vi "Convert From Base64.vi"(8 "error in (no error)":errorcluster, 11 "Base64 String":string) -> (0 "error out":errorcluster, 3 "String":string)   [LabVIEW 2015, in "Front Panel Publisher.lvlib"]
doc: "This VI converts a Base 64 string to its string equivalent. Base64 strings are commonly used in Internet protocols such as HTTP, SMTP, etc."
uses:
  Front Panel Publisher.lvlib
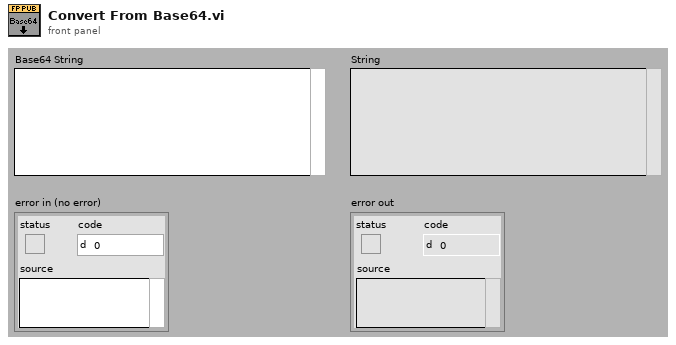
[diagram p1: front panel]
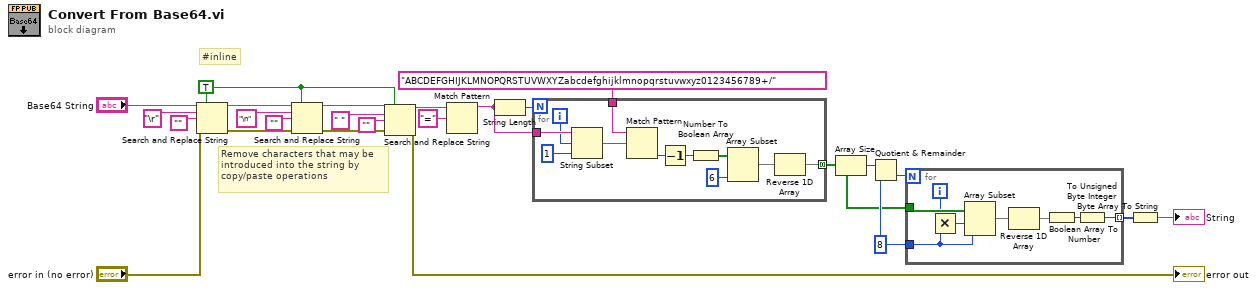
[diagram p0: block diagram]
diagram:
  w25 = TRUE ("replace all? (F)")
  w14 = 8 ("y")
  # "#inline"
  # "Remove characters that may be\nintroduced into the string by\ncopy/paste operations"
  n1 = Search and Replace String(replace all?=w25, input string="Base64 String", search string="\r" ("replace string (\"\")"), replace string="", error in="error in (no error)") -> (result string=w19:string, error out=w6:errorcluster)  [unwired: 5 out]
  n2 = Search and Replace String(replace all?=w25, input string=w19, search string="\n" ("replace string (\"\")"), replace string="", error in=w6) -> (result string=w23:string, error out=w5:errorcluster)  [unwired: 5 out]
  n3 = Search and Replace String(replace all?=w25, input string=w23, search string=" " ("replace string (\"\")"), replace string="", error in=w5) -> (result string=w24:string, error out=→"error out":errorcluster)  [unwired: 5 out]
  n4 = Match Pattern(string=w24, regular expression="=") -> (before substring=w9:string)  [unwired: 4 out]
  n5 = String Length(string=w9) -> (length=w7:i32)
  n6 = for {
    N: w7 -> [_]
    tunnel: w9 -> [w36]
    tunnel: "ABCDEFGHIJKLMNOPQRSTUVWXYZabcdefghijklmnopqrstuvwxyz0123456789+/" -> [w33]
    tunnel: [w26] -> w13 mode=concatenating
    i -> [w34]
    n7 = String Subset(string=w36, offset (0)=w34, length (rest)=1 ("length (rest)")) -> (substring=w32:string)
    n8 = Match Pattern(string=w33, regular expression=w32) -> (offset past match=w31:i32)  [unwired: 4 out]
    n9 = Decrement(x=w31) -> (x-1=w30:i32)
    n10 = Number To Boolean Array(number=w30) -> (Boolean array=w29:bool[])
    n11 = Array Subset(array=w29, length=6) -> (w27:bool[])  [unwired: 1 in]
    n12 = Reverse 1D Array(array=w27) -> (reversed array=w26:bool[])
  }
  n13 = Array Size(array=w13) -> (size(s)=w11:i32)
  n14 = Quotient & Remainder(x=w11, y=w14) -> (floor(x/y)=w12:i32)  [unwired: 1 out]
  n15 = for {
    N: w12 -> [_]
    tunnel: w13 -> [w44]
    tunnel: w14 -> [w43]
    tunnel: [w39] -> w15 mode=indexing
    i -> [w42]
    n16 = Multiply(x=w42, y=w43) -> (x*y=w37:i32)
    n17 = Array Subset(array=w44, index=w37, length=w43) -> (w41:bool[])
    n18 = Reverse 1D Array(array=w41) -> (reversed array=w38:bool[])
    n19 = Boolean Array To Number(Boolean array=w38) -> (number=w40:u32)
    n20 = To Unsigned Byte Integer(number=w40) -> (unsigned 8bit integer=w39:u8)
  }
  n21 = Byte Array To String(unsigned byte array=w15) -> (string=→"String":string)
